vi "3.vi"() -> ()   [LabVIEW 2026]
uses:
  <vilib>/numeric/Random Number (Range) DBL.vi
  3global.vi
panel:
  out "Waveform Graph":dbl[][](graph)
  in  "stop":bool
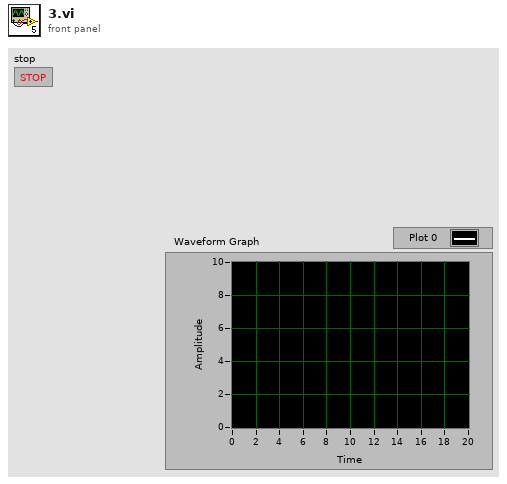
[diagram p1: front panel]
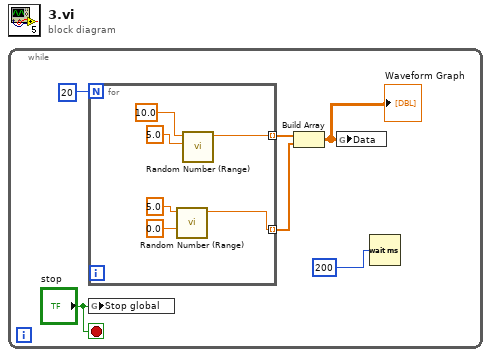
[diagram p0: block diagram]
diagram:
  n1 = while {
    stop <- "stop" stop-if-true
    n2 = for {
      N: 20 -> [_]
      tunnel: [w10] -> w5 mode=indexing
      tunnel: [w7] -> w4 mode=indexing
      n3 = call-poly <vilib>:"Random Number (Range).vi"("lower bound (0)"=0.0, "upper bound (100)"=5.0) -> ("number"=w7:dbl)  [unwired: 9 in]
      n4 = call-poly <vilib>:"Random Number (Range).vi"("lower bound (0)"=5.0, "upper bound (100)"=10.0) -> ("number"=w10:dbl)  [unwired: 9 in]
    }
    n5 = global write "3global.vi" "Stop global"("stop") -> ()
    n6 = Build Array(w5, w4) -> (w2:dbl[][])
    "Waveform Graph" <- w2
    n7 = global write "3global.vi" "Data"(w2) -> ()
    n8 = Wait (ms)(milliseconds to wait=u32 200) -> ()  [unwired: 1 out]
  }
